vi "SNA Strip Channel From Parameters.vi"(4 "Parameters to Measure":T1[](array[typedef]) {"Channel" min=1 max=99 step=1; "Parameter"."Stimulus Port" min=1 step=1; "Parameter"."Response Port" min=1 step=1}) -> (1 "Parameters to Measure":string[](array[string]))   [LabVIEW 2011]
uses:
  tests/S Parameter/TypeDefs/SP Parameter to Measure.ctl
  tests/S Parameter/TypeDefs/SP Parameter.ctl
  tests/S Parameter/TypeDefs/SP Calibration State.ctl
  tests/S Parameter/TypeDefs/SP Measurement Format.ctl
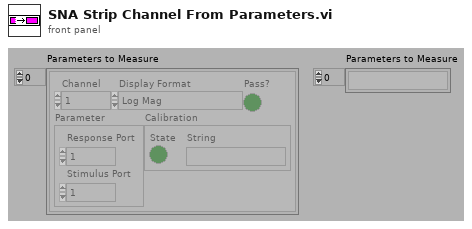
[diagram p1: front panel]
types:
  T1 = typedef "SP Parameter to Measure.ctl" = cluster{"Channel":i8, "Parameter":T2, "Calibration":T3, "Display Format":T4, "Pass?":bool}
  T2 = typedef "SP Parameter.ctl" = cluster{"Stimulus Port":i8, "Response Port":i8}
  T3 = typedef "SP Calibration State.ctl" = cluster{"State":bool, "String":string}
  T4 = typedef "SP Measurement Format.ctl" = enum32{"Log Mag", "Phase", "Delay", "Smith (R+jX)", "Polar (Re/Im)", "Linear Mag", "SWR", "Real", "Imaginary", "Smith (Lin/Phase)", "Smith (Log/Phase)", "Smith (Real/Imag)", "Smith (G+jB)", "Polar (Lin/Phase)", "Polar (Log/Phase)", "Expanded Phase", "Positive Phase", "Inverted Smith", "Unwrapped Phase", "Power Out", "Power In", "Linear Mag/Phase", "Log Mag/Phase", "Real/Imaginary"}
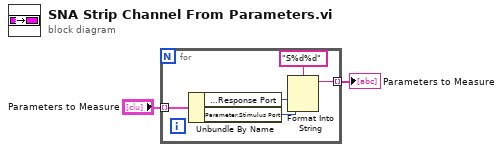
[diagram p0: block diagram]
diagram:
  n1 = for {
    tunnel: "Parameters to Measure" -> [w7] mode=indexing
    tunnel: [w3] -> w1 mode=indexing
    n2 = Unbundle By Name(w7) -> ("Parameter.Response Port"=w6:i8, "Parameter.Stimulus Port"=w5:i8)
    n3 = Format Into String(format string="S%d%d", w6, w5) -> (resulting string=w3:string)  [unwired: 2 in, 1 out]
  }
  "Parameters to Measure" <- w1
